vi "Convert joystick to teleop command.vi"(8 "error in (no error)":errorcluster, 10 "Teleop command in":T1, 11 "Joystick in":refnum<k1>) -> (0 "error out":errorcluster, 2 "Teleop command out":T1, 3 "Joystick out":refnum<k1>)   [LabVIEW 2012]
uses:
  Teleop command.ctl
  <vilib>/Utility/inputDevices.llb/joystickAcquire.vi
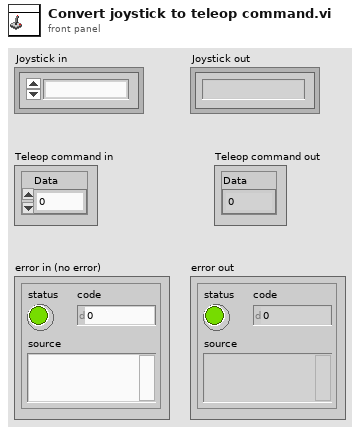
[diagram p1: front panel]
types:
  T1 = typedef "Teleop command.ctl" = cluster{"Data":dbl}
  T2 = cluster{"X axis":i32, "Y axis":i32, "Z axis":i32, "X axis rotation":i32, "Y axis rotation":i32, "Z axis rotation":i32, "U axis":i32, "V axis":i32}
  T3 = cluster{"button 1":bool, "button 2":bool, "button 3":bool, "button 4":bool, "button 5":bool, "button 6":bool, "button 7":bool, "button 8":bool, "button 9":bool, "button 10":bool, "button 11":bool, "button 12":bool, "button 13":bool, "button 14":bool, "button 15":bool, "button 16":bool, "button 17":bool, "button 18":bool, "button 19":bool, "button 20":bool, "button 21":bool, "button 22":bool, "button 23":bool, "button 24":bool, "button 25":bool, "button 26":bool, "button 27":bool, "button 28":bool, "button 29":bool, "button 30":bool, "button 31":bool, "button 32":bool}
  T4 = cluster{"pov 1":i32, "pov 2":i32, "pov 3":i32, "pov 4":i32}
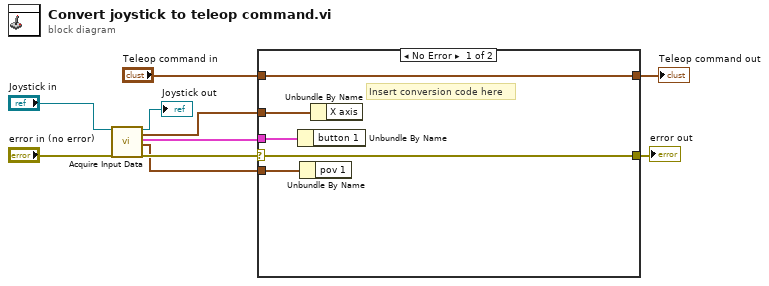
[diagram p0: block diagram]
diagram:
  n1 = call-poly <vilib>:"Acquire Input Data.vi"("device ID"="Joystick in", "error in (no error)"="error in (no error)") -> ("device ID"=→"Joystick out":refnum<k1>, "axis info"=w3:T2, "button info"=w2:T3, "direction info"=w1:T4, "error out"=w7:errorcluster)  [unwired: 13 in]
  n2 = case shown="No Error" w7 {
    selector: w7 -> [w15 w17]
    tunnel: [w15 w17] -> w6
    tunnel: "Teleop command in" -> [w12 w16]
    tunnel: [w12 w16] -> w5
    tunnel: w3 -> [w14 _]
    tunnel: w2 -> [w13 _]
    tunnel: w1 -> [w11 _]
    frame No Error {
      # "Insert conversion code here"
      n3 = Unbundle By Name(w13) -> ()  [unwired: 1 out]
      n4 = Unbundle By Name(w11) -> ()  [unwired: 1 out]
      n5 = Unbundle By Name(w14) -> ()  [unwired: 1 out]
    }
    frame Error {
    }
  }
  "Teleop command out" <- w5
  "error out" <- w6
